vi "Run Test For Data Encapsulation Example.vi"(8 "error in":errorcluster) -> (0 "error out":errorcluster, 1 "result":bool, 2 "time":timestamp)   [LabVIEW 2020]
doc: "This VI pretends to run a test and returns a random pass/fail result and a time stamp."
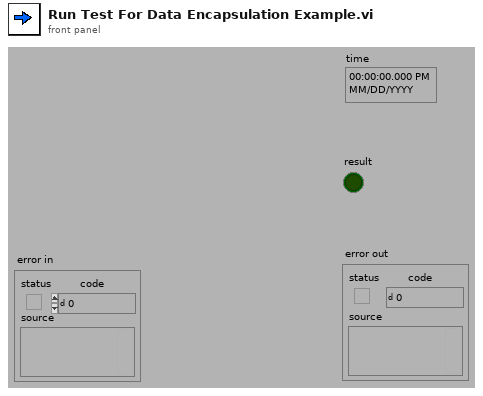
[diagram p1: front panel]
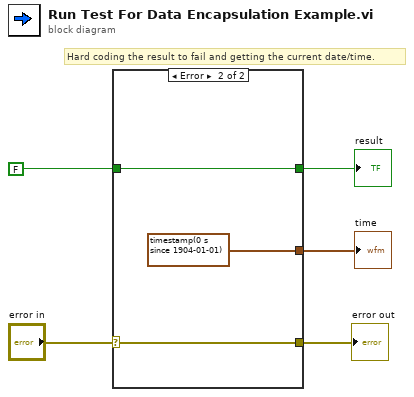
[diagram p0: block diagram]
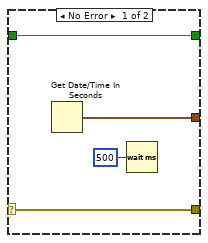
[diagram p2: hidden frame]
diagram:
  # "Hard coding the result to fail and getting the current date/time."
  n1 = case shown="Error" "error in" {
    selector: "error in" -> [w8 w12]
    tunnel: [w8 w12] -> w4
    tunnel: [w6 w10] -> w3
    tunnel: [w7 timestamp(0 s since 1904-01-01) ("seconds since 1Jan1904")] -> w2
    tunnel: FALSE -> [w6 w10]
    frame No Error {
      n2 = Get Date/Time In Seconds() -> (seconds since 1Jan1904=w7:timestamp)
      n3 = Wait (ms)(milliseconds to wait=u32 500) -> ()  [unwired: 1 out]
    }
    frame Error {
    }
  }
  "error out" <- w4
  "result" <- w3
  "time" <- w2
